vi "PIDController_CalculateError_Internal.vi"(11 "in PID_CONTROLLER":T1={"Kp"=0.0, "Ki"=0.0, "Kd"=0.0, "Period"=0.0, "Max_Integral"=0.0, "Min_Integral"=0.0, "Max_Input"=0.0, "Min_Input"=0.0, "Continuous"=FALSE, "PositionError"=0.0, "VelocityError"=0.0, "PrevError"=0.0, "Total_Integral"=0.0, "PositionTolerance"=0.0, "VelocityTolerance"=0.0, "SetPoint"=0.0, "Kf"=0.0, "Prev_Deriv"=0.0, "Prev_Deriv 2"=0.0, "DerivativeFilter"=FALSE, "Min_Output"=-9.99e+35, "Max_Output"=9.9e+35, "Prev_F_P"=0.0, "Prev_F_P_2"=0.0, "AntiWindupActive"=FALSE, "Measurement"=0.0, "IntegralZone"=9.9e+30} {"IntegralZone" format="%16_6e"; "Measurement" format="%16_6e"; "Prev_F_P_2" format="%16_6e"; "Prev_F_P" format="%16_6e"; "Max_Output" format="%16_6e"; "Min_Output" format="%16_6e"; "Prev_Deriv 2" format="%16_6e"; "Prev_Deriv" format="%16_6e"; "Kf" format="%16_6e"; "SetPoint" format="%16_6e"; "VelocityTolerance" format="%16_6e"; "PositionTolerance" format="%16_6e"; "Total_Integral" format="%16_6e"; "PrevError" format="%16_6e"; "VelocityError" format="%16_6e"; "PositionError" format="%16_6e"; "Min_Input" format="%16_6e"; "Max_Input" format="%16_6e"; "Min_Integral" format="%16_6e"; "Max_Integral" format="%16_6e"; "Period" format="%16_6e"; "Kd" format="%16_6e"; "Ki" format="%16_6e"; "Kp" format="%16_6e"}) -> (1 "VelocityError":dbl, 3 "PositionError":dbl)   [LabVIEW 2019, in "Trajectory_Library.lvlib"]
doc: "Internal routine to calculate the position and velocity errors."
uses:
  Trajectory_Library.lvlib
  TypeDef/PID_CONTROLLER.ctl
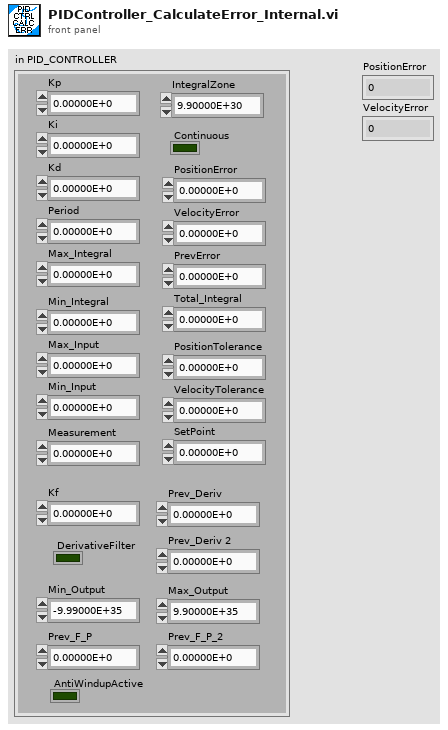
[diagram p1: front panel]
types:
  T1 = typedef "Trajectory_Library.lvlib/PID_CONTROLLER.ctl" = cluster{"Kp":dbl, "Ki":dbl, "Kd":dbl, "Period":dbl, "Max_Integral":dbl, "Min_Integral":dbl, "Max_Input":dbl, "Min_Input":dbl, "Continuous":bool, "PositionError":dbl, "VelocityError":dbl, "PrevError":dbl, "Total_Integral":dbl, "PositionTolerance":dbl, "VelocityTolerance":dbl, "SetPoint":dbl, "Kf":dbl, "Prev_Deriv":dbl, "Prev_Deriv 2":dbl, "DerivativeFilter":bool, "Min_Output":dbl, "Max_Output":dbl, "Prev_F_P":dbl, "Prev_F_P_2":dbl, "AntiWindupActive":bool, "Measurement":dbl, "IntegralZone":dbl}
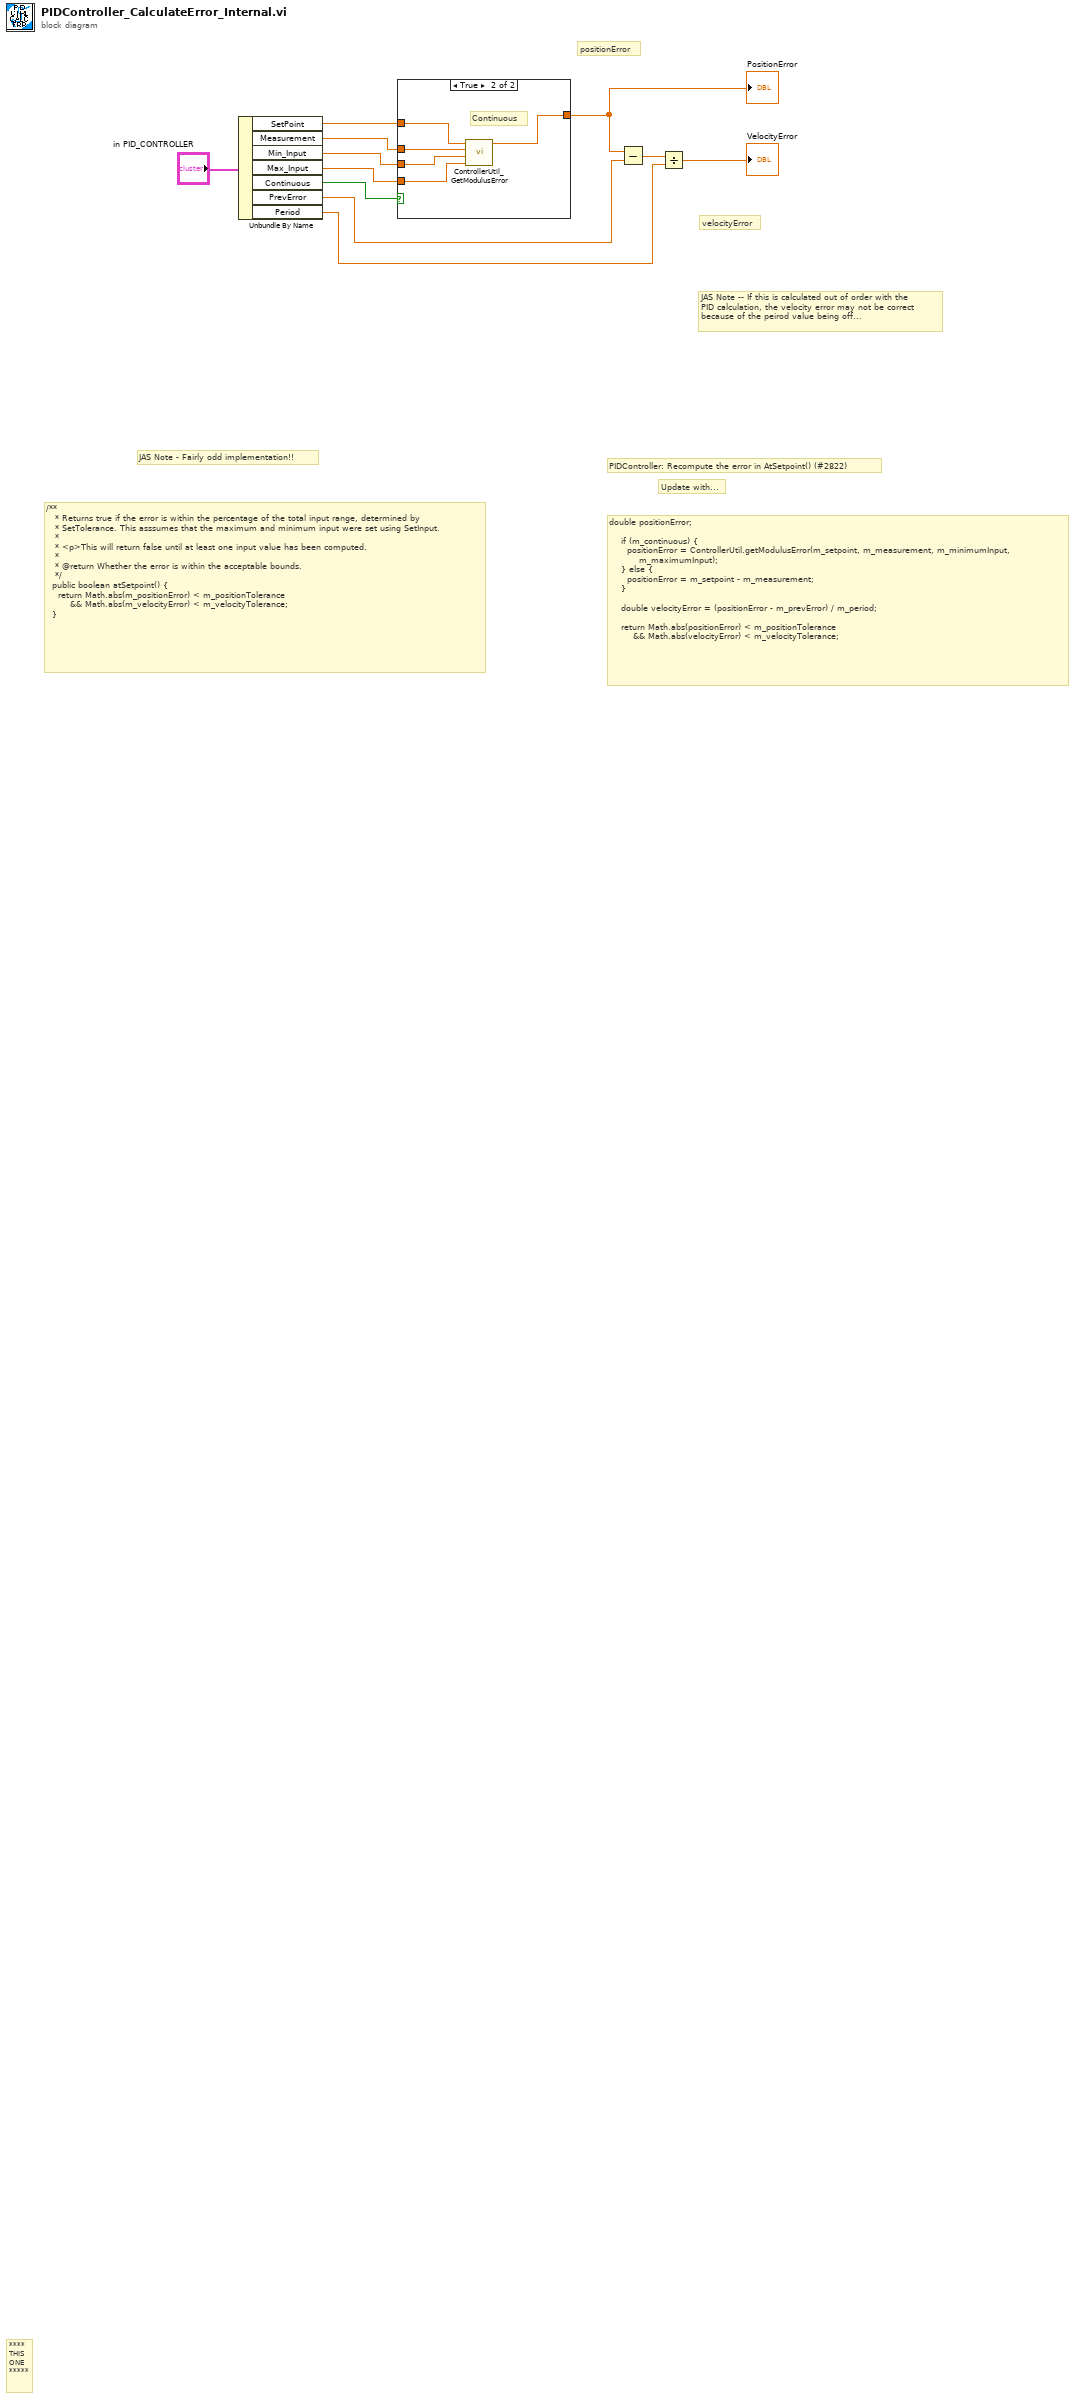
[diagram p0: block diagram]
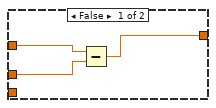
[diagram p2: hidden frame]
diagram:
  # "JAS Note -- If this is calculated out of order with the\nPID calculation, the velocity error may not be correct\nbecause of the peirod value being off..."
  # "velocityError"
  # "positionError"
  # "Update with..."
  # "double positionError;\n\n    if (m_continuous) {\n      positionError = ControllerUtil.getModulusError(m_setpoint, m_measurement, m_minimumInput,\n          m_maximumInput);\n    } else {\n      positionError = m_setpoint - m_measurement;\n    }\n\n    double velocityError = (positionError - m_prevError) / m_period;\n\n    return Math.abs(positionError) < m_positionTolerance\n        && Math.abs(velocityError) < m_velocityTolerance;"
  # "PIDController: Recompute the error in AtSetpoint() (#2822)"
  # "JAS Note - Fairly odd implementation!!"
  # "/**\n   * Returns true if the error is within the percentage of the total input range, determined by\n   * SetTolerance. This asssumes that the maximum and minimum input were set using SetInput.\n   *\n   * <p>This will return false until at least one input value has been computed.\n   *\n   * @return Whether the error is within the acceptable bounds.\n   */\n  public boolean atSetpoint() {\n    return Math.abs(m_positionError) < m_positionTolerance\n        && Math.abs(m_velocityError) < m_velocityTolerance;\n  }"
  # "****\nTHIS\nONE\n*****"
  n1 = Unbundle By Name("in PID_CONTROLLER") -> ("SetPoint"=w10:dbl, "Measurement"=w9:dbl, "Min_Input"=w8:dbl, "Max_Input"=w7:dbl, "Continuous"=w11:bool, "PrevError"=w5:dbl, "Period"=w3:dbl)
  n2 = case shown="True" w11 {
    tunnel: w10 -> [w14 w19]
    tunnel: w9 -> [w13 w18]
    tunnel: [w12 w15] -> w6
    tunnel: w8 -> [_ w17]
    tunnel: w7 -> [_ w16]
    frame False {
      n3 = Subtract(x=w14, y=w13) -> (x-y=w12:dbl)
    }
    frame True {
      # "Continuous"
      n4 = call "ControllerUtil_GetModulusError.vi"("Maximum_Input"=w16, "Minimum_Input"=w17, "Measurerment(PV)"=w18, "Reference(SP)"=w19) -> ("Error"=w15:dbl)  [unwired: 7 in]
    }
  }
  "PositionError" <- w6
  n5 = Subtract(x=w6, y=w5) -> (x-y=w4:dbl)
  n6 = Divide(x=w4, y=w3) -> (x/y=→"VelocityError":dbl)
